vi "Photocell Control Fan.vi"() -> ()   [LabVIEW 2014]
uses:
  <vilib>/LabVIEW Interface for Arduino/LabVIEW Interface for Arduino.lvlib
panel:
  in  "PWM Pin (3) 2":u8=3
  out "Waveform Chart":dbl(graph)
  in  "PWM Pin (3)":u8=3
  in  "VISA resource":refnum<visa-resource-name>
  out "Light Intensity (0 - 100)":dbl(knob) scale=0.0..100.0
  in  "Photo Cell Pin (0)":u8
  in  "?":bool
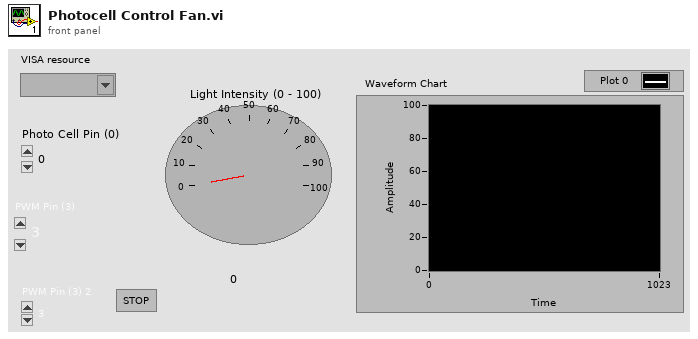
[diagram p1: front panel]
types:
  T1 = typedef "LabVIEW Interface for Arduino.lvlib/Arduino Resource.ctl" = cluster{"VISA resource":refnum<visa-resource-name>, "Board Type":T2, "Connection Type":enum8{"USB / Serial"}, "Bytes Per Packet (15)":u8}
  T2 = typedef "LabVIEW Interface for Arduino.lvlib/Board Type.ctl" = enum16{"Uno", "Dimuelanove w/Atmega 328", "Mega 2560"}
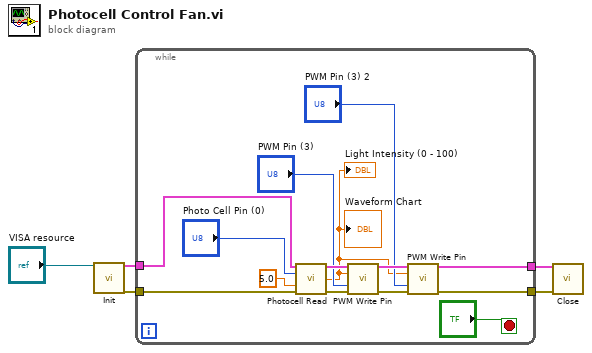
[diagram p0: block diagram]
diagram:
  n1 = call <vilib>:"Init.vi"("VISA resource"="VISA resource") -> ("Arduino Resource"=w5:T1, "error out"=w4:errorcluster)  [unwired: 17 in]
  n2 = while {
    tunnel: w5 -> [w16]
    tunnel: w4 -> [w15]
    tunnel: [w9] -> w3
    tunnel: [w8] -> w2
    stop <- "?" stop-if-true
    n3 = call <vilib>:"Photocell Read.vi"("Arduino Resource"=w16, "Photo Cell Pin (0)"="Photo Cell Pin (0)", "Vcc (5)"=5.0, "error in"=w15) -> ("Arduino Resource"=w13:T1, "Light Intensity (0 - 100)"=w6:dbl, "error out"=w14:errorcluster)  [unwired: 9 in]
    "Light Intensity (0 - 100)" <- w6
    "Waveform Chart" <- w6
    n4 = call <vilib>:"PWM Write Pin.vi"("Arduino Resource"=w13, "Duty Cycle (0 - 255)"=w6, "PWM Pin (3)"="PWM Pin (3)", "error in"=w14) -> ("Arduino Resource"=w11:T1, "error out"=w10:errorcluster)  [unwired: 10 in]
    n5 = call <vilib>:"PWM Write Pin.vi"("Arduino Resource"=w11, "Duty Cycle (0 - 255)"=w6, "PWM Pin (3)"="PWM Pin (3) 2", "error in"=w10) -> ("Arduino Resource"=w9:T1, "error out"=w8:errorcluster)  [unwired: 10 in]
  }
  n6 = call <vilib>:"Close.vi"("Arduino Resource"=w3, "error in"=w2) -> ()  [unwired: 13 in, 1 out]
